vi "PathChoose.vi"(11 "?":T1) -> (3 "Path_Out":path)   [LabVIEW 2017]
uses:
  Ctrls/PathChoose.ctl
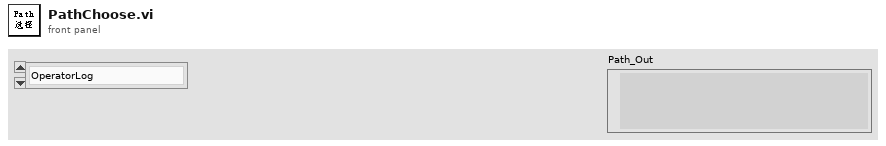
[diagram p1: front panel]
types:
  T1 = typedef "PathChoose.ctl" = enum16{"OperatorLog", "AutoRunLog", "AlmLog", "TestData", "AllTestData", "backup_nvm", "backup_before_flashing"}
  T2 = typedef "TesterInfo.ctl" = cluster{"Station Name":string, "Station Code":string, "ES NO.":string, "Tester ID":string, "PassMark Revision":string, "Rig ID":string, "Deamon_vision":string, "Project Name":string, "FFTesterPath":path, "Enable_User":bool, "Mode":enum16{"682"}, "MES":bool}
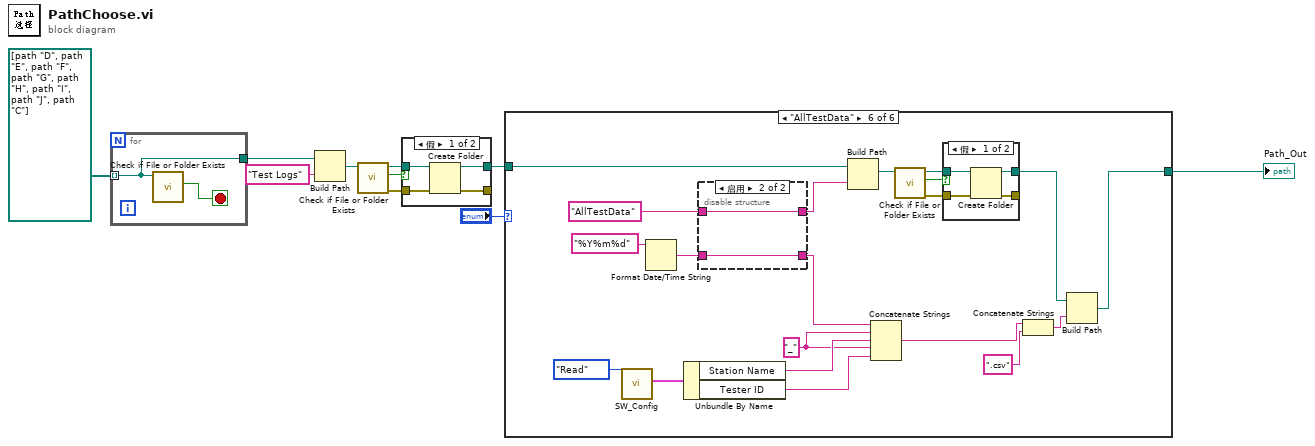
[diagram p0: block diagram]
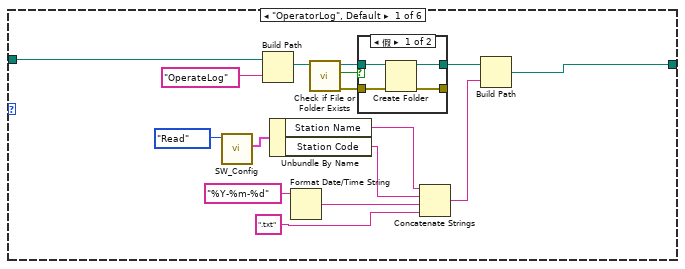
[diagram p2: hidden frame]
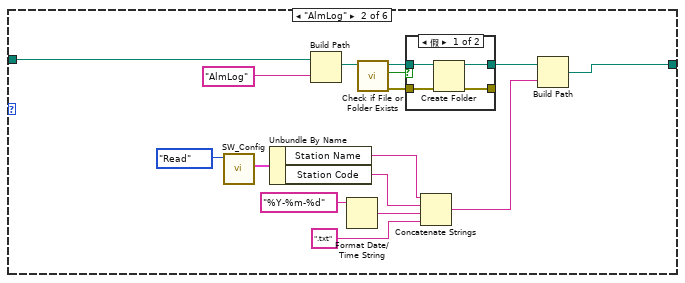
[diagram p4: hidden frame]
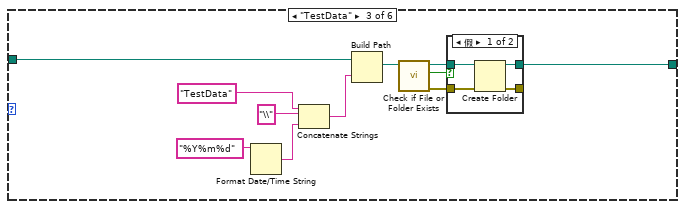
[diagram p6: hidden frame]
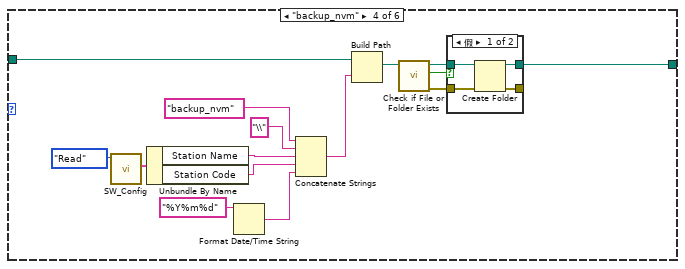
[diagram p8: hidden frame]
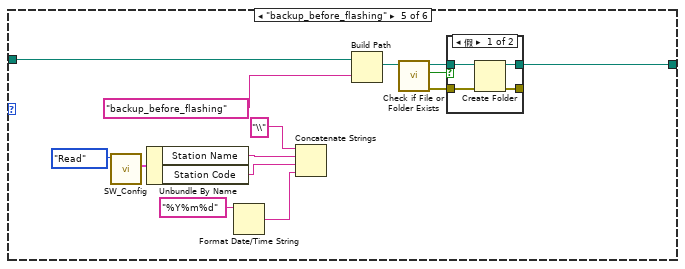
[diagram p10: hidden frame]
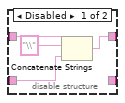
[diagram p12: hidden frame]
diagram:
  n1 = for {
    tunnel: path[] [path "D:/", path "E:/", path "F:/", path "G:/", path "H:/", path "I:/", path "J:/", path "C:/"] -> [w11] mode=indexing
    tunnel: [w11] -> w4
    stop <- w12 stop-if-true
    n2 = call <vilib>:"Check if File or Folder Exists.vi"("path"=w11) -> ("file or folder exists?"=w12:bool)  [unwired: 8 in, 2 out]
  }
  n3 = Build Path(base path=w4, name or relative path="Test Logs") -> (appended path=w2:path)
  n4 = call <vilib>:"Check if File or Folder Exists.vi"("path"=w2) -> ("error out"=w9:errorcluster, "file or folder exists?"=w10:bool, "dup path"=w8:path)  [unwired: 8 in]
  n5 = case shown="假" w10 {
    tunnel: w9 -> [w15 w17]
    tunnel: w8 -> [w16 w18]
    tunnel: [w13 w18] -> w7
    tunnel: [w14 w17] -> _
    frame False {
      n6 = Create Folder(path (use dialog)=w16, error in=w15) -> (created path=w13:path, error out=w14:errorcluster)  [unwired: 1 in, 1 out]
    }
    frame True {
    }
  }
  n7 = case shown="\"AllTestData\"" "?" {
    tunnel: w7 -> [w34 w56 w73 w94 w114 w140]
    tunnel: [w33 w55 w68 w89 w109 w128] -> w1
    frame "OperatorLog", Default {
      n8 = call "SW_Config.vi"("Step"=enum16{"Initial", "Write", "Read"}."Read") -> ("SW Config out"=w19:T2)  [unwired: 9 in, 1 out]
      n9 = Build Path(base path=w34, name or relative path="OperateLog" ("OPfilename")) -> (appended path=w28:path)
      n10 = Unbundle By Name(w19) -> ("Station Name"=w25:string, "Station Code"=w24:string)
      n11 = Format Date/Time String(time format string (%c)="%Y-%m-%d" ("时间格式字符串(%c)")) -> (date/time string=w26:string)  [unwired: 2 in]
      n12 = call <vilib>:"Check if File or Folder Exists.vi"("path"=w28) -> ("error out"=w30:errorcluster, "file or folder exists?"=w29:bool, "dup path"=w31:path)  [unwired: 8 in]
      n13 = case shown="假" w29 {
        tunnel: w30 -> [w37 w39]
        tunnel: w31 -> [w38 w40]
        tunnel: [w35 w40] -> w27
        tunnel: [w36 w39] -> _
        frame False {
          n14 = Create Folder(path (use dialog)=w38, error in=w37) -> (created path=w35:path, error out=w36:errorcluster)  [unwired: 1 in, 1 out]
        }
        frame True {
        }
      }
      n15 = Concatenate Strings(w25, w24, w26, ".txt" ("字符串")) -> (w20:string)
      n16 = Build Path(base path=w27, name or relative path=w20) -> (appended path=w33:path)
    }
    frame "AlmLog" {
      n17 = call "SW_Config.vi"("Step"=enum16{"Initial", "Write", "Read"}."Read") -> ("SW Config out"=w41:T2)  [unwired: 9 in, 1 out]
      n18 = Unbundle By Name(w41) -> ("Station Name"=w43:string, "Station Code"=w42:string)
      n19 = Build Path(base path=w56, name or relative path="AlmLog" ("名称或相对路径")) -> (appended path=w50:path)
      n20 = Format Date/Time String(time format string (%c)="%Y-%m-%d" ("时间格式字符串(%c)")) -> (date/time string=w48:string)  [unwired: 2 in]
      n21 = call <vilib>:"Check if File or Folder Exists.vi"("path"=w50) -> ("error out"=w52:errorcluster, "file or folder exists?"=w51:bool, "dup path"=w53:path)  [unwired: 8 in]
      n22 = case shown="假" w51 {
        tunnel: w52 -> [w59 w61]
        tunnel: w53 -> [w60 w62]
        tunnel: [w57 w62] -> w46
        tunnel: [w58 w61] -> _
        frame False {
          n23 = Create Folder(path (use dialog)=w60, error in=w59) -> (created path=w57:path, error out=w58:errorcluster)  [unwired: 1 in, 1 out]
        }
        frame True {
        }
      }
      n24 = Concatenate Strings(w43, w42, w48, ".txt" ("字符串")) -> (w45:string)
      n25 = Build Path(base path=w46, name or relative path=w45) -> (appended path=w55:path)
    }
    frame "TestData" {
      n26 = Format Date/Time String(time format string (%c)="%Y%m%d") -> (date/time string=w67:string)  [unwired: 2 in]
      n27 = Concatenate Strings("TestData" ("名称或相对路径"), "\\" ("字符串"), w67) -> (w63:string)
      n28 = Build Path(base path=w73, name or relative path=w63) -> (appended path=w69:path)
      n29 = call <vilib>:"Check if File or Folder Exists.vi"("path"=w69) -> ("error out"=w71:errorcluster, "file or folder exists?"=w70:bool, "dup path"=w72:path)  [unwired: 8 in]
      n30 = case shown="假" w70 {
        tunnel: w71 -> [w76 w78]
        tunnel: w72 -> [w77 w79]
        tunnel: [w74 w79] -> w68
        tunnel: [w75 w78] -> _
        frame False {
          n31 = Create Folder(path (use dialog)=w77, error in=w76) -> (created path=w74:path, error out=w75:errorcluster)  [unwired: 1 in, 1 out]
        }
        frame True {
        }
      }
    }
    frame "backup_nvm" {
      n32 = call "SW_Config.vi"("Step"=enum16{"Initial", "Write", "Read"}."Read") -> ("SW Config out"=w84:T2)  [unwired: 9 in, 1 out]
      n33 = Unbundle By Name(w84) -> ("Station Name"=w82:string, "Station Code"=w81:string)
      n34 = Format Date/Time String(time format string (%c)="%Y%m%d") -> (date/time string=w80:string)  [unwired: 2 in]
      n35 = Concatenate Strings("backup_nvm" ("名称或相对路径"), "\\" ("字符串"), w82, w81, w80) -> (w85:string)
      n36 = Build Path(base path=w94, name or relative path=w85) -> (appended path=w90:path)
      n37 = call <vilib>:"Check if File or Folder Exists.vi"("path"=w90) -> ("error out"=w92:errorcluster, "file or folder exists?"=w91:bool, "dup path"=w93:path)  [unwired: 8 in]
      n38 = case shown="假" w91 {
        tunnel: w92 -> [w97 w99]
        tunnel: w93 -> [w98 w100]
        tunnel: [w95 w100] -> w89
        tunnel: [w96 w99] -> _
        frame False {
          n39 = Create Folder(path (use dialog)=w98, error in=w97) -> (created path=w95:path, error out=w96:errorcluster)  [unwired: 1 in, 1 out]
        }
        frame True {
        }
      }
    }
    frame "backup_before_flashing" {
      n40 = call "SW_Config.vi"("Step"=enum16{"Initial", "Write", "Read"}."Read") -> ("SW Config out"=w106:T2)  [unwired: 9 in, 1 out]
      n41 = Unbundle By Name(w106) -> ("Station Name"=w104:string, "Station Code"=w103:string)
      n42 = Format Date/Time String(time format string (%c)="%Y%m%d") -> (date/time string=w102:string)  [unwired: 2 in]
      n43 = Concatenate Strings("\\" ("字符串"), w104, w103, w102) -> ()  [unwired: 1 out]
      n44 = Build Path(base path=w114, name or relative path="backup_before_flashing" ("名称或相对路径")) -> (appended path=w110:path)
      n45 = call <vilib>:"Check if File or Folder Exists.vi"("path"=w110) -> ("error out"=w112:errorcluster, "file or folder exists?"=w111:bool, "dup path"=w113:path)  [unwired: 8 in]
      n46 = case shown="假" w111 {
        tunnel: w112 -> [w117 w119]
        tunnel: w113 -> [w118 w120]
        tunnel: [w115 w120] -> w109
        tunnel: [w116 w119] -> _
        frame False {
          n47 = Create Folder(path (use dialog)=w118, error in=w117) -> (created path=w115:path, error out=w116:errorcluster)  [unwired: 1 in, 1 out]
        }
        frame True {
        }
      }
    }
    frame "AllTestData" {
      w123 = "_" ("字符串")
      n48 = call "SW_Config.vi"("Step"=enum16{"Initial", "Write", "Read"}."Read") -> ("SW Config out"=w127:T2)  [unwired: 9 in, 1 out]
      n49 = Format Date/Time String(time format string (%c)="%Y%m%d") -> (date/time string=w133:string)  [unwired: 2 in]
      n50 = Unbundle By Name(w127) -> ("Station Name"=w126:string, "Tester ID"=w125:string)
      n51 = disable-structure shown="启用" {
        disable-tunnel: "AllTestData" ("名称或相对路径") -> [w144 w146]
        disable-tunnel: w133 -> [w143 w145]
        disable-tunnel: [w141 w146] -> w132
        disable-tunnel: [_ w145] -> w121
        frame Disabled {
          n52 = Concatenate Strings(w144, "\\" ("字符串"), w143) -> (w141:string)
        }
        frame Enabled {
        }
      }
      n53 = Build Path(base path=w140, name or relative path=w132) -> (appended path=w136:path)
      n54 = Concatenate Strings(w121, w123, w126, w123, w125) -> (w122:string)
      n55 = call <vilib>:"Check if File or Folder Exists.vi"("path"=w136) -> ("error out"=w138:errorcluster, "file or folder exists?"=w137:bool, "dup path"=w139:path)  [unwired: 8 in]
      n56 = case shown="假" w137 {
        tunnel: w138 -> [w149 w151]
        tunnel: w139 -> [w150 w152]
        tunnel: [w147 w152] -> w129
        tunnel: [w148 w151] -> _
        frame False {
          n57 = Create Folder(path (use dialog)=w150, error in=w149) -> (created path=w147:path, error out=w148:errorcluster)  [unwired: 1 in, 1 out]
        }
        frame True {
        }
      }
      n58 = Concatenate Strings(w122, ".csv" ("string")) -> (w131:string)
      n59 = Build Path(base path=w129, name or relative path=w131) -> (appended path=w128:path)
    }
  }
  "Path_Out" <- w1
